vi "AUTON_Unpack.vi"(0 "all rows":dbl[][](array[numeric]), 5 "Index":i32) -> (4 "Primitive ID":i16, 6 "Desired Heading":dbl, 8 "Time/Distance":dbl, 10 "Power":dbl, 12 "Indexer Speed":dbl, 13 "Shooter Setpoint":dbl, 14 "Harvester Speed":dbl, 15 "Shooter Speed":dbl)   [LabVIEW 2012]
doc: "Use this VI to separate the autonomous array data into individual arrays. First array is Primitive ID, second is heading, etc."
panel:
  out "Misc 2":dbl
  out "Misc 1":dbl
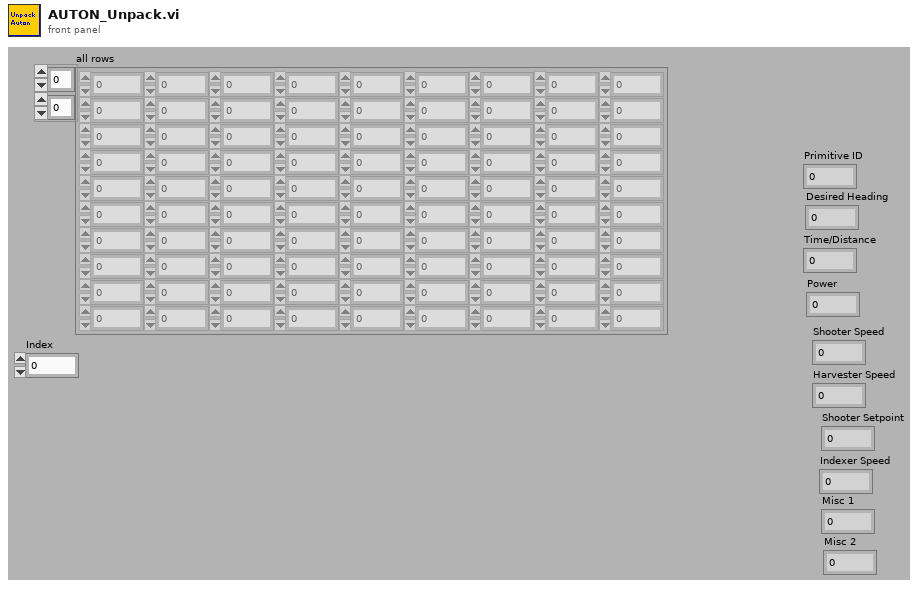
[diagram p1: front panel]
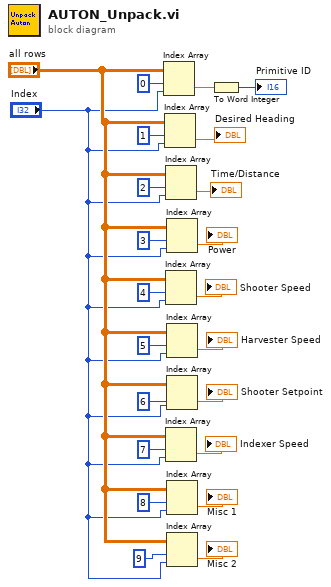
[diagram p0: block diagram]
diagram:
  n1 = Index Array(array="all rows", index (row)=0, index (col)="Index") -> (element=w20:dbl)
  n2 = Index Array(array="all rows", index (row)=1, index (col)="Index") -> (element=→"Desired Heading":dbl)
  n3 = Index Array(array="all rows", index (row)=2, index (col)="Index") -> (element=→"Time/Distance":dbl)
  n4 = Index Array(array="all rows", index (row)=4, index (col)="Index") -> (element=→"Shooter Speed":dbl)
  n5 = Index Array(array="all rows", index (row)=7, index (col)="Index") -> (element=→"Indexer Speed":dbl)
  n6 = Index Array(array="all rows", index (row)=3, index (col)="Index") -> (element=→"Power":dbl)
  n7 = Index Array(array="all rows", index (row)=5, index (col)="Index") -> (element=→"Harvester Speed":dbl)
  n8 = Index Array(array="all rows", index (row)=6, index (col)="Index") -> (element=→"Shooter Setpoint":dbl)
  n9 = Index Array(array="all rows", index (row)=8, index (col)="Index") -> (element=→"Misc 1":dbl)
  n10 = Index Array(array="all rows", index (row)=9, index (col)="Index") -> (element=→"Misc 2":dbl)
  n11 = To Word Integer(number=w20) -> (16bit integer=→"Primitive ID":i16)
